vi "FL Implication Max.vi"(5 "user MF interpolating polynomials":T1[](array[typedef]) {"coa_x(y) coeff" format="%.4g"; "Area(y) coeff" format="%.4g"; "X(y) coeff" format="%.4g"; "Y(x) coeff" format="%.4g"; "Y" format="%.4g"; "X" format="%.4g"}, 6 "user-defined \nshape index":i32, 7 "Function":T2=10 items=["Triangle", "Trapezoid", "Singleton", "Sigmoid", "Gaussian", "User-Defined"], 9 "Weight":dbl, 10 "Implication":T3 items=["Minimum", "Product"], 11 "Points (X)":dbl[](array[numeric])) -> (1 "X(Max)":dbl, 2 "X(Max) product":dbl)   [LabVIEW 2017, in "NI_Fuzzy_Logic_API.lvlib"]
uses:
  <vilib>/addons/Fuzzy Logic/NI_Fuzzy_Logic_API.lvlib
  <vilib>/addons/Fuzzy Logic/TypeDefs/FL Consequent Implication.ctl
  <vilib>/addons/Fuzzy Logic/TypeDefs/FL Membership Function Shape.ctl
  <vilib>/addons/Fuzzy Logic/TypeDefs/FL Interpolating polynomials.ctl
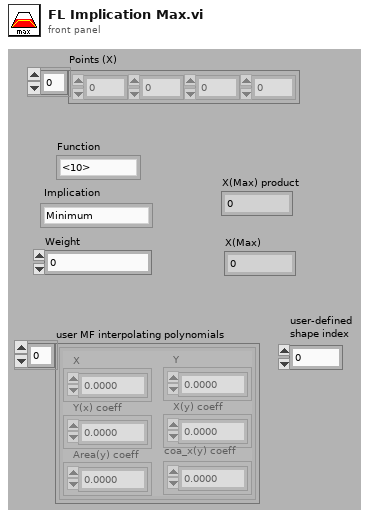
[diagram p1: front panel]
types:
  T1 = typedef "NI_Fuzzy_Logic_API.lvlib/FL Interpolating polynomials.ctl" = cluster{"X":dbl[], "Y":dbl[], "Y(x) coeff":dbl[][], "X(y) coeff":dbl[][], "Area(y) coeff":dbl[][], "coa_x(y) coeff":dbl[][]}
  T2 = typedef "NI_Fuzzy_Logic_API.lvlib/FL Membership Function Shape.ctl" = u16
  T3 = typedef "NI_Fuzzy_Logic_API.lvlib/FL Consequent Implication.ctl" = u16
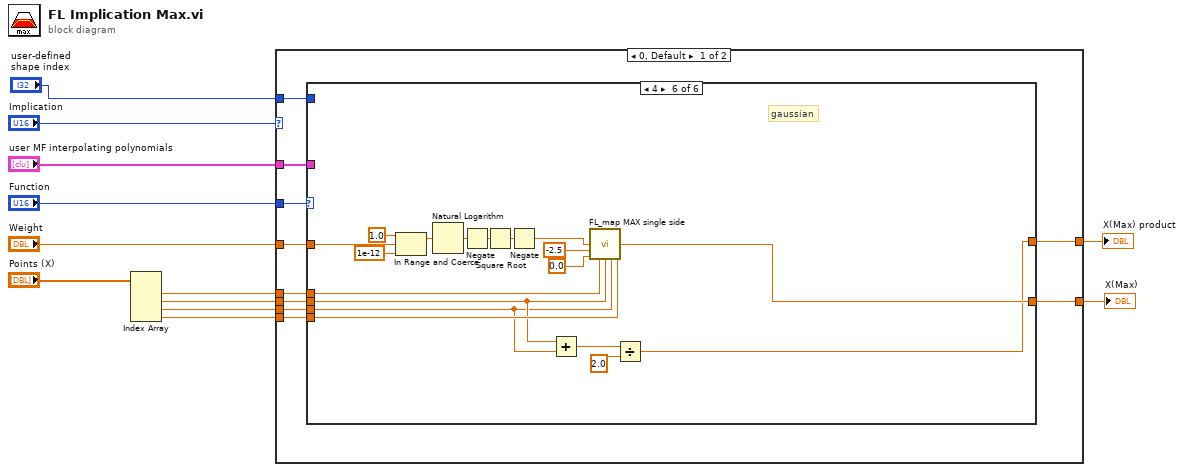
[diagram p0: block diagram]
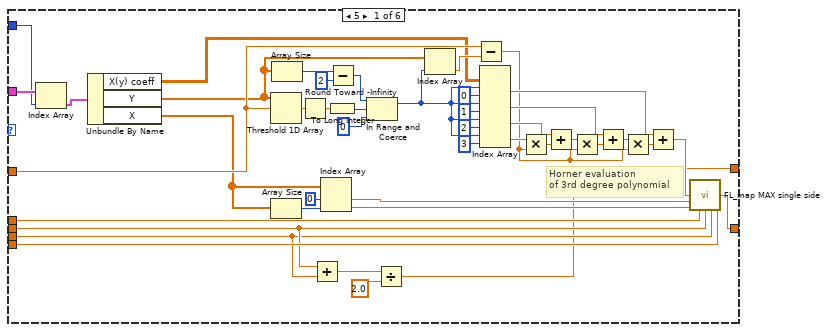
[diagram p2: hidden frame]
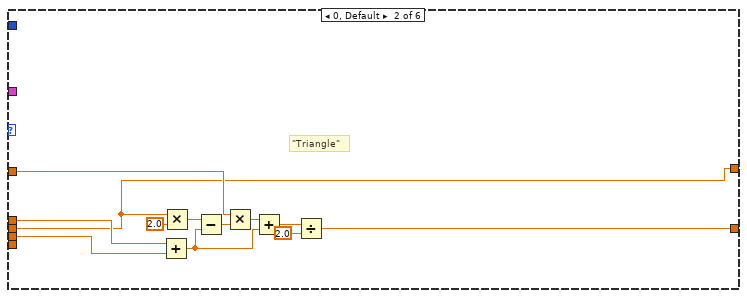
[diagram p3: hidden frame]
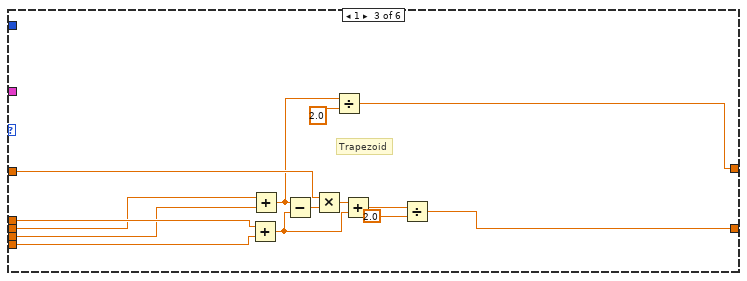
[diagram p4: hidden frame]
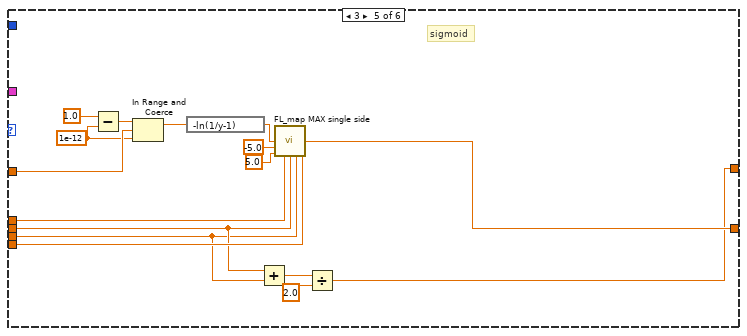
[diagram p6: hidden frame]
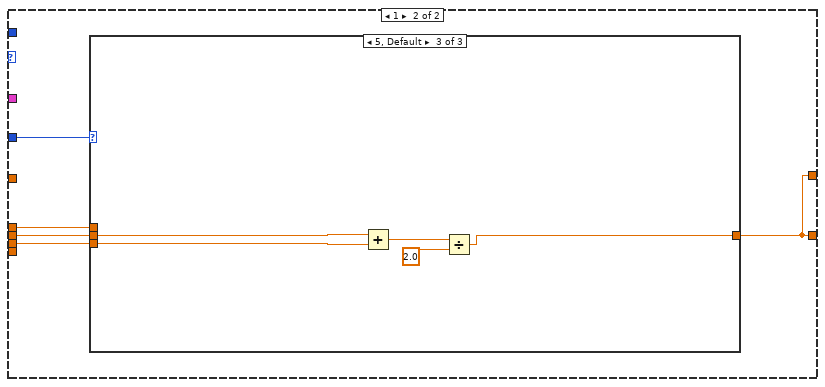
[diagram p7: hidden frame]
diagram:
  n1 = Index Array(array="Points (X)") -> (element #1=w8:dbl, element #2=w7:dbl, element #3=w6:dbl, element #4=w5:dbl)  [unwired: 4 in]
  n2 = case shown="0, Default" "Implication" {
    tunnel: "Function" -> [w22 w128]
    tunnel: "Weight" -> [w21 _]
    tunnel: "user MF interpolating polynomials" -> [w20 _]
    tunnel: w8 -> [w19 w127]
    tunnel: w7 -> [w18 w131]
    tunnel: w6 -> [w17 w130]
    tunnel: w5 -> [w16 _]
    tunnel: [w15 w129] -> w4
    tunnel: [w14 w129] -> w2
    tunnel: "user-defined \nshape index" -> [w13 _]
    frame 0, Default {
      n3 = case shown="4" w22 {
        tunnel: w21 -> [w32 w72 w86 _ w102 w112]
        tunnel: [w62 w67 w83 w92 w101 w120] -> w15
        tunnel: w19 -> [w64 w77 w85 w92 w108 w126]
        tunnel: w18 -> [w26 w66 w84 _ w104 w122]
        tunnel: w17 -> [w25 w76 w81 _ w103 w121]
        tunnel: w16 -> [w63 _ w82 _ w107 w125]
        tunnel: w20 -> [w65 _ _ _ _ _]
        tunnel: [w24 w66 w78 w92 w100 w119] -> w14
        tunnel: w13 -> [w23 _ _ _ _ _]
        frame 5 {
          # "Horner evaluation\nof 3rd degree polynomial"
          n4 = Index Array(array=w65, index=w23) -> (element=w60:T1)
          n5 = Unbundle By Name(w60) -> ("X(y) coeff"=w30:dbl[][], "Y"=w31:dbl[], "X"=w29:dbl[])
          n6 = Threshold 1D Array(2:w32, 3:w31) -> (0:w39:dbl)  [unwired: 1 out]
          n7 = Array Size(array=w29) -> (size(s)=w59:i32)
          n8 = Array Size(array=w31) -> (size(s)=w36:i32)
          n9 = Round Toward -Infinity(1:w39) -> (0:w40:dbl)
          n10 = Add(x=w26, y=w25) -> (x+y=w28:dbl)
          n11 = Index Array(array=w29, index #1=0 ("index"), index #2=w59) -> (element #1=w58:dbl, element #2=w57:dbl)
          n12 = To Long Integer(number=w40) -> (32bit integer=w41:i32)
          n13 = Subtract(x=w36, y=2) -> (x-y=w35:i32)
          n14 = In Range and Coerce(upper limit=w35, x=w41, lower limit=0) -> (coerced(x)=w43:i32)  [unwired: 1 out]
          n15 = Divide(x=w28, y=2.0) -> (x/y=w24:dbl)
          n16 = Index Array(array=w31, index=w43) -> (element=w38:dbl)
          n17 = Subtract(x=w32, y=w38) -> (x-y=w34:dbl)
          n18 = Index Array(array=w30, index (row) #1=w43, index (col) #1=0 ("disabled index (col)"), index (row) #2=w43, index (col) #2=1 ("disabled index (col)"), index (row) #3=w43, index (col) #3=2 ("disabled index (col)"), index (row) #4=w43, index (col) #4=3 ("disabled index (col)")) -> (element #1=w56:dbl, element #2=w53:dbl, element #3=w50:dbl, element #4=w48:dbl)
          n19 = Multiply(x=w48, y=w34) -> (x*y=w49:dbl)
          n20 = Add(x=w50, y=w49) -> (x+y=w51:dbl)
          n21 = Multiply(x=w51, y=w34) -> (x*y=w52:dbl)
          n22 = Add(x=w53, y=w52) -> (x+y=w54:dbl)
          n23 = Multiply(x=w54, y=w34) -> (x*y=w55:dbl)
          n24 = Add(x=w56, y=w55) -> (x+y=w33:dbl)
          n25 = call <vilib>:"FL_map MAX single side.vi"("X(Max)"=w33, "x_l"=w58, "x_r"=w57, "x0"=w64, "x1"=w26, "x2"=w25, "x3"=w63) -> ("X(Max)"=w62:dbl)  [unwired: 1 in, 7 out]
        }
        frame 0, Default {
          # "\"Triangle\""
          n26 = Add(x=w77, y=w76) -> (x+y=w70:dbl)
          n27 = Multiply(x=w66, y=2.0) -> (x*y=w74:dbl)
          n28 = Subtract(x=w74, y=w70) -> (x-y=w73:dbl)
          n29 = Multiply(x=w72, y=w73) -> (x*y=w71:dbl)
          n30 = Add(x=w71, y=w70) -> (x+y=w69:dbl)
          n31 = Divide(x=w69, y=2.0) -> (x/y=w67:dbl)
        }
        frame 1 {
          # "Trapezoid"
          n32 = Add(x=w85, y=w82) -> (x+y=w89:dbl)
          n33 = Add(x=w84, y=w81) -> (x+y=w79:dbl)
          n34 = Subtract(x=w79, y=w89) -> (x-y=w87:dbl)
          n35 = Multiply(x=w86, y=w87) -> (x*y=w88:dbl)
          n36 = Divide(x=w79, y=2.0) -> (x/y=w78:dbl)
          n37 = Add(x=w88, y=w89) -> (x+y=w90:dbl)
          n38 = Divide(x=w90, y=2.0) -> (x/y=w83:dbl)
        }
        frame 2 {
          # "singleton"
        }
        frame 3 {
          w95 = 1e-12 ("lower limit")
          # "sigmoid"
          n39 = Subtract(x=1.0, y=w95) -> (x-y=w94:dbl)
          n40 = In Range and Coerce(upper limit=w94, x=w102, lower limit=w95) -> (coerced(x)=w93:dbl)  [unwired: 1 out]
          n41 = expression code="-ln(1/y-1)"(w93) -> (w99:dbl)
          n42 = Add(x=w104, y=w103) -> (x+y=w106:dbl)
          n43 = call <vilib>:"FL_map MAX single side.vi"("X(Max)"=w99, "x_l"=-5.0, "x_r"=5.0, "x0"=w108, "x1"=w104, "x2"=w103, "x3"=w107) -> ("X(Max)"=w101:dbl)  [unwired: 2 in, 6 out]
          n44 = Divide(x=w106, y=2.0) -> (x/y=w100:dbl)
        }
        frame 4 {
          # "gaussian"
          n45 = In Range and Coerce(upper limit=1.0, x=w112, lower limit=1e-12) -> (coerced(x)=w109:dbl)  [unwired: 1 out]
          n46 = Natural Logarithm(1:w109) -> (0:w117:dbl)
          n47 = Negate(x=w117) -> (-x=w116:dbl)
          n48 = Square Root(x=w116) -> (sqrt(x)=w118:dbl)
          n49 = Negate(x=w118) -> (-x=w115:dbl)
          n50 = Add(x=w122, y=w121) -> (x+y=w124:dbl)
          n51 = call <vilib>:"FL_map MAX single side.vi"("X(Max)"=w115, "x_l"=-2.5, "x_r"=0.0, "x0"=w126, "x1"=w122, "x2"=w121, "x3"=w125) -> ("X(Max)"=w120:dbl)  [unwired: 1 in, 7 out]
          n52 = Divide(x=w124, y=2.0) -> (x/y=w119:dbl)
        }
      }
    }
    frame 1 {
      n53 = case shown="5, Default" w128 {
        tunnel: w131 -> [w132 _ w138]
        tunnel: w130 -> [_ _ w137]
        tunnel: [w132 w133 w134] -> w129
        tunnel: w127 -> [_ w133 _]
        frame 0 {
        }
        frame 2 {
        }
        frame 5, Default {
          n54 = Add(x=w138, y=w137) -> (x+y=w136:dbl)
          n55 = Divide(x=w136, y=2.0) -> (x/y=w134:dbl)
        }
      }
    }
  }
  "X(Max)" <- w4
  "X(Max) product" <- w2
